vi "Wrap.vi"(9 "Max y":sgl, 10 "Max x":sgl, 11 "Vector 2D in":refnum<class "Vector 2D.lvclass">) -> (3 "Vector 2D out":refnum<class "Vector 2D.lvclass">)   [LabVIEW 2021, in "Vector 2D.lvclass"]
uses:
  Vector 2D.lvclass
  Vector 2D.lvclass/Vector 2D.ctl
  Math/Math.lvlib
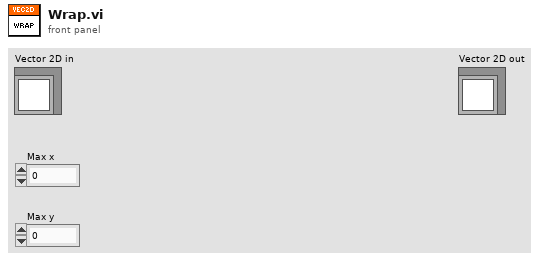
[diagram p1: front panel]
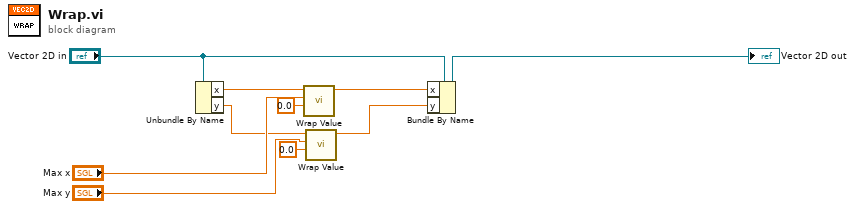
[diagram p0: block diagram]
diagram:
  n1 = Unbundle By Name("Vector 2D in") -> ("x"=w6:sgl, "y"=w3:sgl)
  n2 = call "Wrap Value.vi"("Min"=sgl 0.0, "Max"="Max x", "Value"=w6) -> ("Wrapped Value"=w1:sgl)  [unwired: 8 in]
  n3 = call "Wrap Value.vi"("Min"=sgl 0.0, "Max"="Max y", "Value"=w3) -> ("Wrapped Value"=w2:sgl)  [unwired: 8 in]
  n4 = Bundle By Name(cluster="Vector 2D in", "x"=w1, "y"=w2) -> (→"Vector 2D out":refnum<class "Vector 2D.lvclass">)
